vi "XY Graph Get Max Legend Size.vi"(8 "Error In":errorcluster, 10 "Default (8)":i32=8, 11 "XYGraph Refnum":T1) -> (0 "Error Out":errorcluster, 1 "Max Legend Size Found?":bool, 2 "Max Legend Size":i32=8, 3 "XYGraph Refnum":T1)   [LabVIEW 2019, in "XY Graph Add-Ons.lvlib"]
uses:
  XY Graph Add-Ons.lvlib
  XY Graph Refnum.ctl
  XY Graph Property Tag List.ctl
  <vilib>/UserTags/UserTags.lvlib
  Variant/Variant to Data/Variant to Data.lvlib
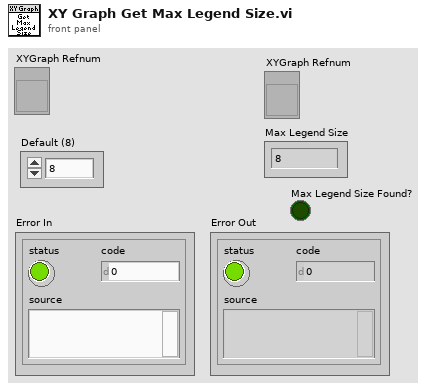
[diagram p1: front panel]
types:
  T1 = typedef "XY Graph Add-Ons.lvlib/XY Graph Refnum.ctl" = refnum<vi>
  T2 = typedef "XY Graph Add-Ons.lvlib/XY Graph Property Tag List.ctl" = enum16{"Max Legend Size", "Preserved Plots", "XScales.GridColors", "YScales.GridColors", "TipStrip String", "TipStrip Visible", "Tool Panels Visibility", "Plots Metadata"}
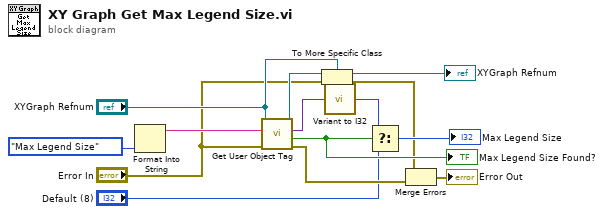
[diagram p0: block diagram]
diagram:
  n1 = Format Into String(XY_Graph_Property_Tag_List."Max Legend Size" ("XY Graph Property Tag")) -> (resulting string=w4:string)  [unwired: 3 in, 1 out]
  n2 = call <vilib>:"Get User Object Tag.vi"("error in (no error)"="Error In", "Tag Name"=w4, "Generic Refnum"="XYGraph Refnum") -> ("error out"=w14:errorcluster, "Was Tag Found?"=w10:bool, "Value"=w13:variant, "dup Generic Refnum"=w8:refnum<vi>)  [unwired: 5 in]
  "Max Legend Size Found?" <- w10
  n3 = To More Specific Class(target class="XYGraph Refnum", reference=w8, error in="Error In") -> (specific class reference=→"XYGraph Refnum":T1, error out=w1:errorcluster)
  n4 = call "Variant to I32.vi"("Variant"=w13) -> ("Value"=w12:i32)  [unwired: 8 in]
  n5 = Select(t=w12, s=w10, f="Default (8)") -> (s? t:f=→"Max Legend Size":i32)
  n6 = Merge Errors(w1, w14) -> (→"Error Out":errorcluster)
